vi "Path Fiducials with No Empty Paths.vi"(11 "Path Fiducials":T6(array[cluster])) -> (3 "Path Fiducials (no empty paths)":T6(array[cluster]))   [LabVIEW 2011]
uses:
  Shared Components/Utils/Type Definitions/Part Fiducials.ctl
  Shared Components/Utils/Type Definitions/Fiducial Image.ctl
  Shared Components/Vec3d Class/Vec3d Class.lvclass
  Shared Components/Utils/Type Definitions/Physical Image.ctl
  <vilib>/vision/Image Controls.llb/IMAQ Image.ctl
  Shared Components/Utils/Type Definitions/Fiducial with Source.ctl
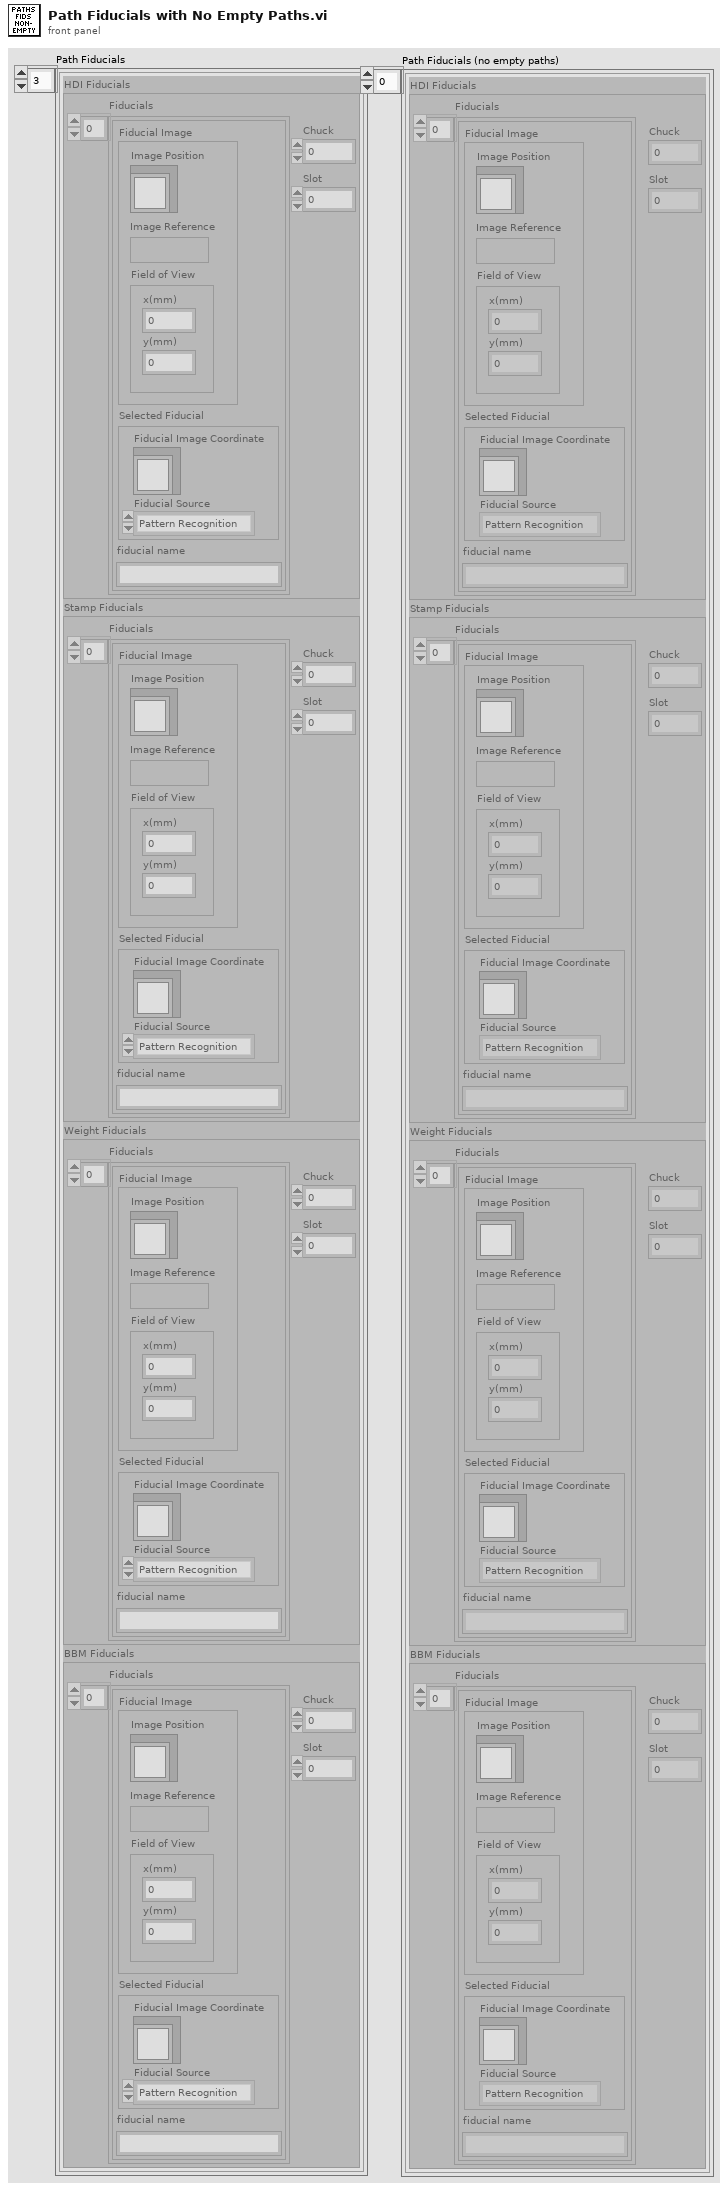
[diagram p1: front panel]
types:
  T1 = typedef "Part Fiducials.ctl" = cluster{"Fiducials":T2[], "Chuck":i32, "Slot":i32}
  T2 = typedef "Fiducial Image.ctl" = cluster{"Fiducial Image":T3, "Selected Fiducial":T5, "fiducial name":string}
  T3 = typedef "Physical Image.ctl" = cluster{"Image Position":refnum<class "Vec3d Class.lvclass">, "Image Reference":T4, "Field of View":cluster{"x(mm)":dbl, "y(mm)":dbl}}
  T4 = typedef "IMAQ Image.ctl" = refnum<image>
  T5 = typedef "Fiducial with Source.ctl" = cluster{"Fiducial Image Coordinate":refnum<class "Vec3d Class.lvclass">, "Fiducial Source":enum16{"Pattern Recognition", "User", "Error", "Default"}}
  T6 = cluster{"HDI Fiducials":T1, "Stamp Fiducials":T1, "Weight Fiducials":T1, "BBM Fiducials":T1}[]
  T7 = cluster{"HDI Fiducials":T1, "Stamp Fiducials":T1, "Weight Fiducials":T1, "BBM Fiducials":T1}
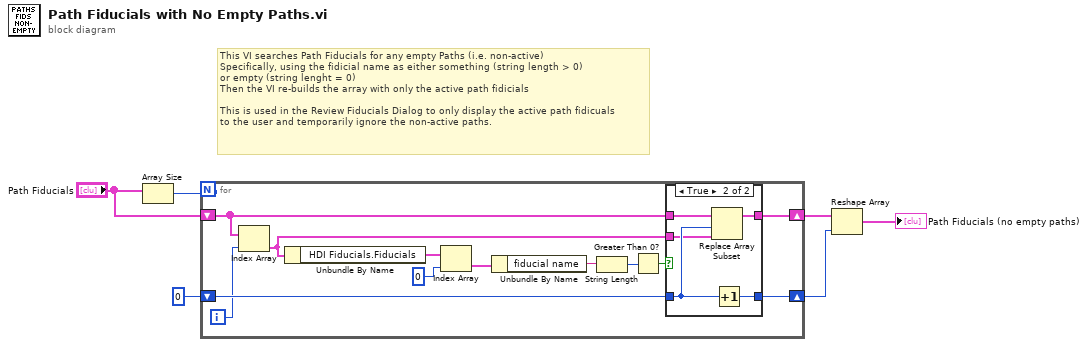
[diagram p0: block diagram]
diagram:
  # "This VI searches Path Fiducials for any empty Paths (i.e. non-active)\nSpecifically, using the fidicial name as either something (string length > 0)\nor empty (string lenght = 0)\nThen the VI re-builds the array with only the active path fidicials\n\nThis is used in the Review Fiducials Dialog to only display the active path fidicuals\nto the user and temporarily ignore the non-active paths."
  n1 = Array Size(array="Path Fiducials") -> (size(s)=w6:i32)
  n2 = for {
    N: w6 -> [_]
    shift-right: [w15] -> w2
    shift-left: 0 -> [w16]
    shift-right: [w14] -> w3
    shift-left: "Path Fiducials" -> [w13]
    i -> [w12]
    n3 = Index Array(array=w13, index=w12) -> (element=w7:T7)
    n4 = Unbundle By Name(w7) -> ("HDI Fiducials.Fiducials"=w11:T2[])
    n5 = Index Array(array=w11, index=0) -> (element=w9:T2)
    n6 = Unbundle By Name(w9) -> ("fiducial name"=w8:string)
    n7 = String Length(string=w8) -> (length=w18:i32)
    n8 = Greater Than 0?(x=w18) -> (x > 0?=w17:bool)
    n9 = case shown="True" w17 {
      tunnel: w13 -> [w20 w23]
      tunnel: w16 -> [w19 w22]
      tunnel: [w19 w25] -> w15
      tunnel: [w20 w24] -> w14
      tunnel: w7 -> [_ w21]
      frame False {
      }
      frame True {
        n10 = Replace Array Subset(array=w23, new element=w21, index=w22) -> (w24:T6)
        n11 = Increment(x=w22) -> (x+1=w25:i32)
      }
    }
  }
  n12 = Reshape Array(w3, w2) -> (→"Path Fiducials (no empty paths)":T6)
